vi "drawCrosshairs_v2.000.vi"(8 "error in (no error)":errorcluster, 10 "pipette tip location (px)":i32[](array[numeric]), 11 "image in":T1(plugin-control) caption="Slice view in") -> (0 "error out":errorcluster, 3 "image out":T1(plugin-control) caption="Slice view out")   [LabVIEW 2015]
panel:
  in  "circle diameter (px)":i32=30
  # "drawCrosshairs_v2.000"
  # "draws a crosshair on image"
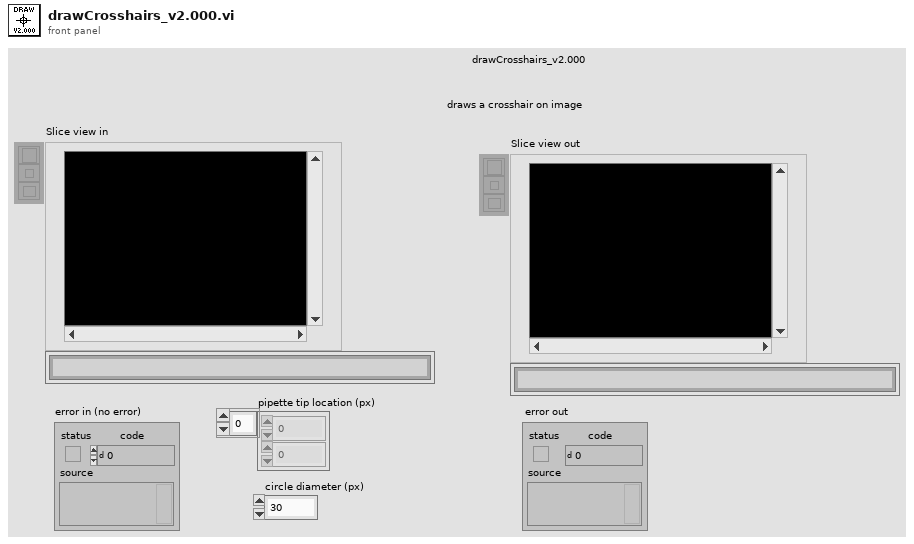
[diagram p1: front panel]
types:
  T1 = typedef "IMAQ Image.ctl" = refnum<image>
  T2 = cluster{"Left":i32, "Top":i32, "Right":i32, "Bottom":i32}
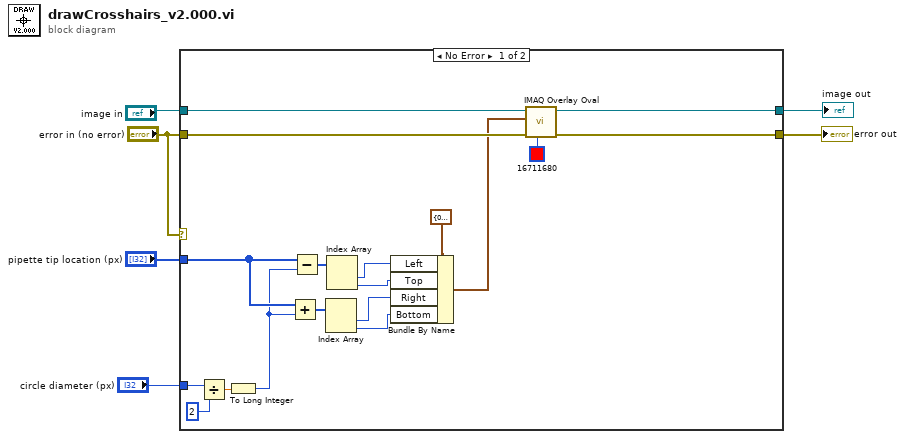
[diagram p0: block diagram]
diagram:
  n1 = case shown="No Error" "error in (no error)" {
    tunnel: "image in" -> [w24 w26]
    tunnel: "error in (no error)" -> [w23 w25]
    tunnel: [w21 w26] -> w5
    tunnel: [w20 w25] -> w4
    tunnel: "pipette tip location (px)" -> [w14 _]
    tunnel: "circle diameter (px)" -> [w10 _]
    frame No Error {
      n2 = Divide(x=w10, y=2) -> (x/y=w8:dbl)
      n3 = To Long Integer(number=w8) -> (32bit integer=w7:i32)
      n4 = Add(x=w14, y=w7) -> (x+y=w17:i32[])
      n5 = Subtract(x=w14, y=w7) -> (x-y=w13:i32[])
      n6 = Index Array(array=w17) -> (element #1=w16:i32, element #2=w15:i32)  [unwired: 2 in]
      n7 = Index Array(array=w13) -> (element #1=w12:i32, element #2=w11:i32)  [unwired: 2 in]
      n8 = Bundle By Name(cluster=T2 {"Left"=0, "Top"=0, "Right"=0, "Bottom"=0} ("Bounding Rectangle"), "Left"=w12, "Top"=w11, "Right"=w16, "Bottom"=w15) -> (w18:T2)
      n9 = call "IMAQ Overlay Oval"("Color"=u32 16711680, "error in (no error)"=w23, "Bounding Rectangle"=w18, "Image"=w24) -> ("error out"=w20:errorcluster, "Image Out"=w21:T1)  [unwired: 6 in]
    }
    frame Error {
    }
  }
  "image out" <- w5
  "error out" <- w4
